vi "ImportCSV.vi"(11 "Settings in":T1={"Name of test"="", "Date"=timestamp(0 s since 1904-01-01), "Location"="", "Template"="", "Soundcard"="", "resolution"=32, "Sampling rate"=48000, "Ch1 Gain "=25.0, "Ch2 Gain"=10.0, "Sample time (s)"=0.3, "Pre-trigger (s)"=0.01, "Hammer Threshold"=10.0, "Positions"=12, "Taps/Position"=5, "Set Names"="", "Freq resolution"=10.0, "Hammer cutoff"=0.0, "Mic cutoff"=0.0, "Double bounce "=0.0, "Hammer Cal"=10.0, "dB Offset"=0.0, "Accel Cal"=10.0, "Vibrometer Cal"=0.0, "Mic Cal"=0.0, "Output"=2, "Voltage Cal"=1.0, "Vibrometer Port"="ASRL27::INSTR", "Range"=4, "High Pass"=2, "Bandwidth"=4, "X Range"=[], "Y Range"=[], "dB Spread"=0.0, "Trigger"=0, "Ch_1"=25, "Ch_2"=25, "flip?"=FALSE, "60Hz"=FALSE, "Time offset"=0.0, "Piezo Cal"=1.0, "Default Notes"=""} {"Ch_2" min=1 step=1; "Ch_1" min=1 max=100 step=1; "Trigger" items=["Hammer (force)", "Self-tap", "Spacebar"]; "Bandwidth" items=["1 kHz"=1, "5 kHz"=5, "10 kHz"=10, "25 kHz"=25, "50 kHz"=50, "100 kHz"=100]; "High Pass" items=["Off", "13 Hz", "104 Hz"]; "Range" items=["10 mm/s"=1, "20 mm/s"=2, "50 mm/s"=5, "100 mm/s"=10, "200 mm/s"=20, "500 mm/s"=50, "1 m/s"=100, "2 m/s"=200]; "Output" items=["Accelerometer", "Speed (from acceleration)", "Microphone", "Vibrometer", "Piezo"]; "Voltage Cal" format="%#_13g"; "Ch2 Gain" format="%#_13g"; "Ch1 Gain" format="%#_13g"; "Double bounce" min=0.0; "Mic cutoff" min=0.0 format="%#_4g"; "Hammer cutoff" min=0.0 format="%#_4g"; "Freq resolution" min=0.0; "Pre-trigger (s)" format="%#_13g"; "Date" format="%<%H:%M\n%d/%m/%y>T"; "resolution" items=["16 bit"=16, "24 bit"=24, "32 bit"=32]; "Sampling rate" items=["22050 samp/s"=22050, "44100 samp/s"=44100, "48000 samp/s"=48000]}) -> ()   [LabVIEW 2022 SP3]
uses:
  PreferencesControl.ctl
  <vilib>/Utility/error.llb/Trim Whitespace One-Sided.vi
panel:
  out "trf":cluster{dbl, dbl, cdb[]}[](array[cluster])
  in  "Tab Control":enum32{"Intro", "Params", "Settings", "Saving"}(tab)
  in  "delimiter":u16(ring) items=["tab", "comma"]
  in  "Save Button":bool
  in  "Instrument Name":string(combo)
  in  "CSV Path":path
  out "FRF":cluster{"x0":dbl, "df":dbl, dbl[]}[](graph)
  out "text":string
  in  "skip first N lines":i32=1
  in  "Back":bool
  out "Slide":u8(slide) scale=0.0..100.0
  out "Info":string
  # "Welcome To The CSV Translator"
  # "This will translate a csv file into the Obie format"
  # "1. Select a file\nHit the folder button or drag a file on"
  # "2. Translate the data\nMake sure the data looks good\n(I assume that the data is evenly sampled\nand that column 1 is time, 2 is real component of pressure\n3 is the complex component, 4 is time, 5 is real,...)"
  # "3. Save as an instrument\nAdd to an existing or create a new instrument"
  # "4. Repeat or Close\nOpen a new file or close the window"
  # "Hz"
  # "dB"
  # "dB"
  # "sec"
  # "sec"
  # "mV/Pa"
  # "mV/m/s2"
  # "mV/mm/s"
  # "V/N"
  # "sec"
  # "sec"
  # "mV/N"
  # "a.u."
  # "a.u."
  # "sec"
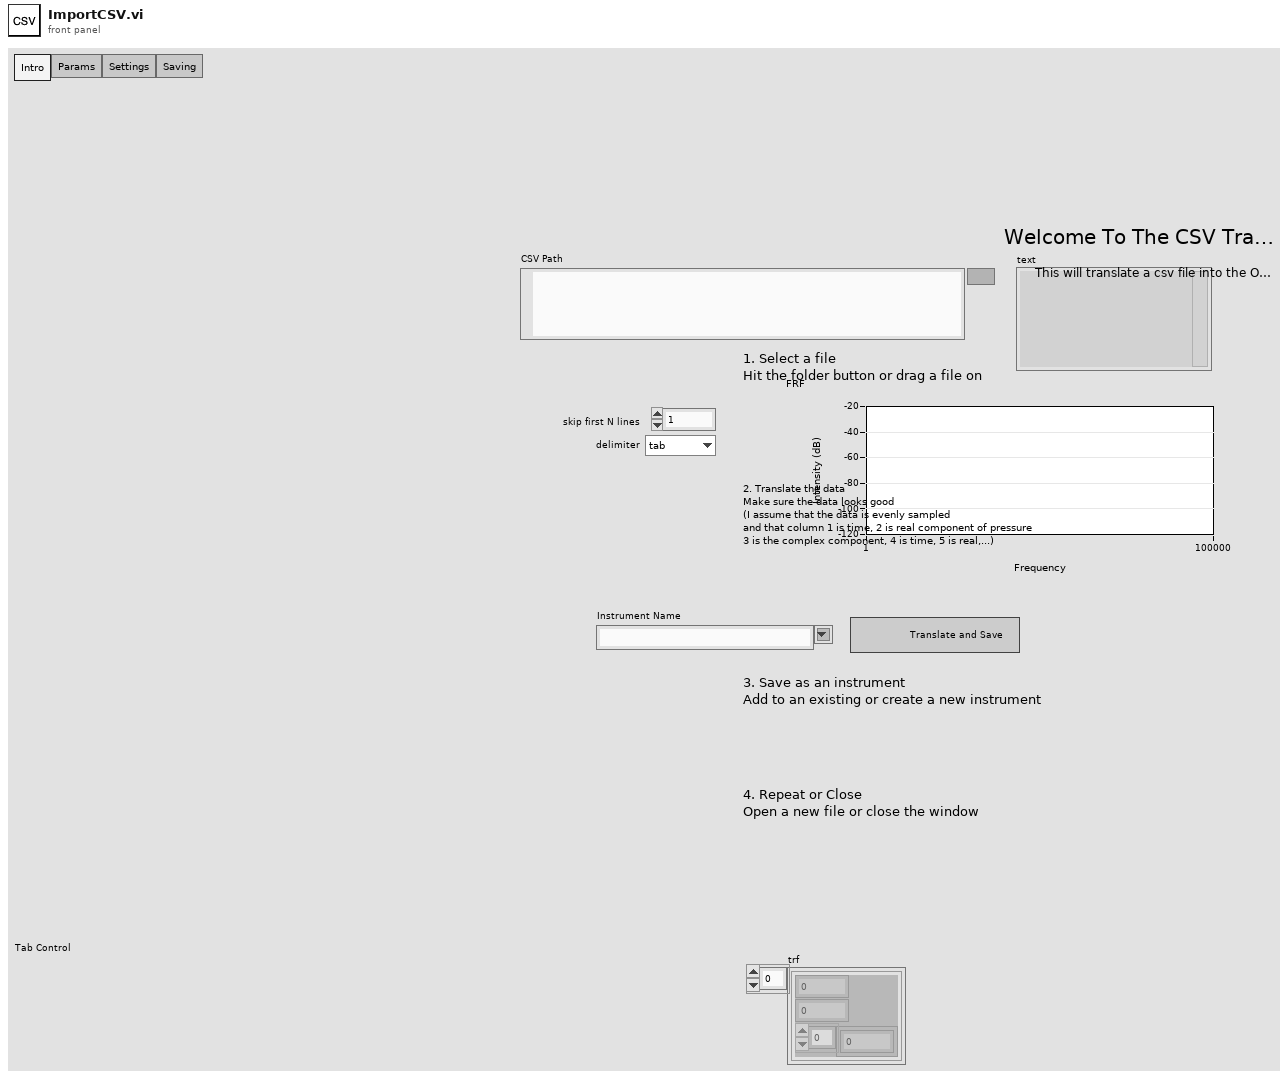
[diagram p1: front panel]
types:
  T1 = typedef "PreferencesControl.ctl" = cluster{"Name of test":string, "Date":timestamp, "Location":string, "Template":string, "Soundcard":string, "resolution":u16, "Sampling rate":u16, "Ch1 Gain ":dbl, "Ch2 Gain":dbl, "Sample time (s)":dbl, "Pre-trigger (s)":dbl, "Hammer Threshold":dbl, "Positions":i16, "Taps/Position":i16, "Set Names":string, "Freq resolution":dbl, "Hammer cutoff":dbl, "Mic cutoff":dbl, "Double bounce ":dbl, "Hammer Cal":dbl, "dB Offset":dbl, "Accel Cal":dbl, "Vibrometer Cal":dbl, "Mic Cal":dbl, "Output":u16, "Voltage Cal":dbl, "Vibrometer Port":refnum<visa-resource-name>, "Range":u16, "High Pass":u16, "Bandwidth":u16, "X Range":cluster{"Minimum":dbl, "Maximum":dbl, "Increment":dbl, "Minor Increment":dbl, "Start":dbl}[], "Y Range":cluster{"Minimum":dbl, "Maximum":dbl, "Increment":dbl, "Minor Increment":dbl, "Start":dbl}[], "dB Spread":dbl, "Trigger":u16, "Ch_1":u8, "Ch_2":u8, "flip?":bool, "60Hz":bool, "Time offset":dbl, "Piezo Cal":dbl, "Default Notes":string}
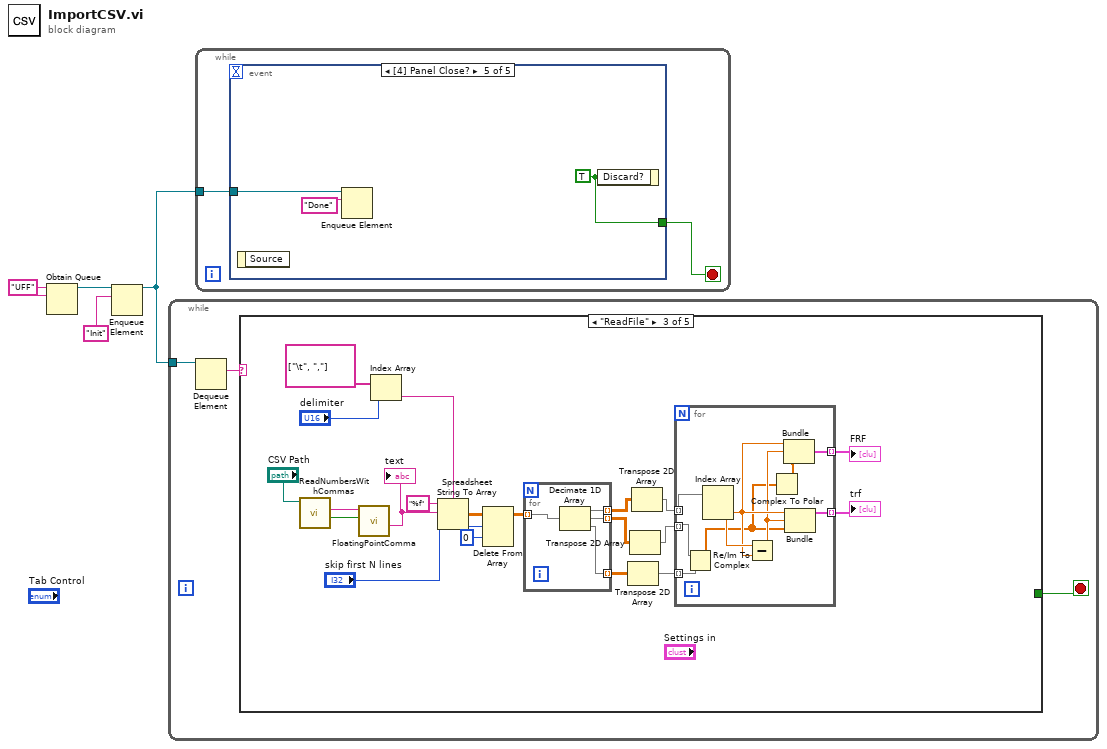
[diagram p0: block diagram]
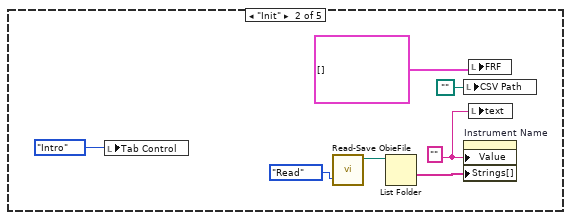
[diagram p3: hidden frame]
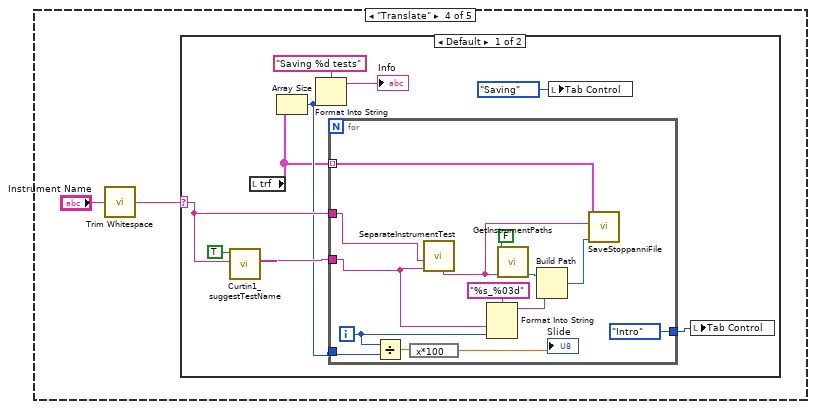
[diagram p4: hidden frame]
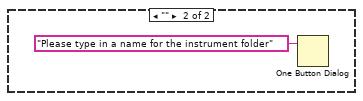
[diagram p5: hidden frame]
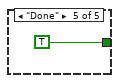
[diagram p6: hidden frame]
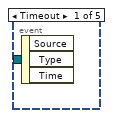
[diagram p7: hidden frame]
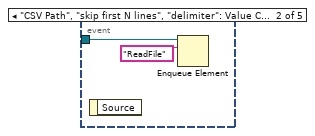
[diagram p8: hidden frame]
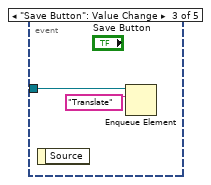
[diagram p9: hidden frame]
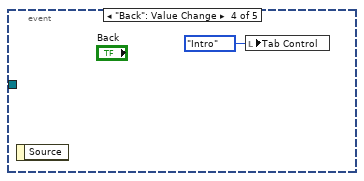
[diagram p10: hidden frame]
diagram:
  w4 = "UFF" ("name (unnamed)")
  n1 = Obtain Queue(name (unnamed)=w4, element data type=w4) -> (queue out=w1:refnum<queue>)  [unwired: 3 in, 2 out]
  n2 = Enqueue Element(queue=w1, element="Init") -> (queue out=w2:refnum<queue>)  [unwired: 2 in, 2 out]
  n3 = while {
    tunnel: w2 -> [w7]
    stop <- w5 stop-if-true
    n4 = Dequeue Element(queue=w7) -> (element=w6:string)  [unwired: 2 in, 3 out]
    n5 = case shown="\"ReadFile\"" w6 {
      tunnel: [_ _ _ _ TRUE ("Discard?")] -> w5
      frame Default {
      }
      frame "Init" {
        w10 = "" ("Value (Signaling)")
        n6 = local write "Tab Control"(enum32{"Intro", "Params", "Settings"}."Intro" ("Tab Control")) -> ()
        n7 = call "Read-Save ObieFile.vi"("Task"=enum16{"Save", "Read"}."Read") -> ("DataPath Out"=w12:path)  [unwired: 8 in, 2 out]
        n8 = List Folder(path=w12) -> (folder names=w11:string[])  [unwired: 3 in, 3 out]
        n9 = local write "CSV Path"(path "" ("CSV Path")) -> ()
        n10 = property on="Instrument Name" class="CmbBox"("Value"=w10, "Strings[]"=w11) -> ()  [unwired: 2 in, 2 out]
        n11 = local write "FRF"(cluster{"x0":dbl, "df":dbl, dbl[]}[] [] ("FRF")) -> ()
        n12 = local write "text"(w10) -> ()
      }
      frame "ReadFile" {
        n13 = call "ReadNumbersWithCommas.vi"("file (use dialog)"="CSV Path") -> ("comma?"=w15:bool, "text"=w17:string)  [unwired: 7 in, 2 out]
        n14 = call "FloatingPointComma.vi"("Comma?"=w15, "String In"=w17) -> ("fixed"=w16:string)  [unwired: 8 in, 1 out]
        "text" <- w16
        n15 = Index Array(array=string[] ["\t", ","], index="delimiter") -> (element=w22:string)
        n16 = Spreadsheet String To Array(delimiter (Tab)=w22, format string="%f", spreadsheet string=w16) -> (array=w33:dbl[][])  [unwired: 1 in]
        n17 = Delete From Array(array=w33, length="skip first N lines", index (row)=0) -> (array with subset deleted=w27:dbl[][])  [unwired: 1 in, 1 out]
        n18 = for {
          tunnel: w27 -> [w48] mode=indexing
          tunnel: [w47] -> w32 mode=indexing
          tunnel: [w46] -> w31 mode=indexing
          tunnel: [w45] -> w21 mode=indexing
          n19 = Decimate 1D Array(w48) -> (w47:dbl[], w46:dbl[], w45:dbl[])
        }
        n20 = Transpose 2D Array(2D array=w21) -> (transposed array=w20:dbl[][])
        n21 = Transpose 2D Array(2D array=w31) -> (transposed array=w29:dbl[][])
        n22 = Transpose 2D Array(2D array=w32) -> (transposed array=w30:dbl[][])
        n23 = for {
          tunnel: w30 -> [w43] mode=indexing
          tunnel: w29 -> [w40] mode=indexing
          tunnel: [w44] -> w28 mode=indexing
          tunnel: w20 -> [w41] mode=indexing
          tunnel: [w37] -> w19 mode=indexing
          n24 = Re/Im To Complex(1:w41, 2:w40) -> (0:w36:cdb[])
          n25 = Index Array(array=w43) -> (element #1=w39:dbl, element #2=w42:dbl)  [unwired: 2 in]
          n26 = Subtract(x=w42, y=w39) -> (x-y=w38:dbl)
          n27 = Complex To Polar(r * e^(i*theta)=w36) -> (r=w35:dbl[])  [unwired: 1 out]
          n28 = Bundle(w39, w38, w35) -> (w37:cluster{dbl, dbl, dbl[]})  [unwired: 1 in]
          n29 = Bundle(w39, w38, w36) -> (w44:cluster{dbl, dbl, cdb[]})  [unwired: 1 in]
        }
        "FRF" <- w19
        "trf" <- w28
      }
      frame "Translate" {
        n30 = call <vilib>:"Trim Whitespace.vi"("string"="Instrument Name") -> ("trimmed string"=w49:string)  [unwired: 1 in]
        n31 = case shown="Default" w49 {
          selector: w49 -> [w58 _]
          frame Default {
            n32 = call "Curtin1_suggestTestName.vi"("instrument"=w58, "Build?"=TRUE) -> ("Suggested Test"=w56:string)  [unwired: 9 in]
            n33 = local read "trf"() -> (w51:cluster{dbl, dbl, cdb[]}[])
            n34 = Array Size(array=w51) -> (size(s)=w54:i32)
            n35 = Format Into String(format string="Saving %d tests", w54) -> (resulting string=→"Info":string)  [unwired: 2 in, 1 out]
            n36 = for {
              tunnel: w58 -> [w69]
              tunnel: w56 -> [w66]
              tunnel: w54 -> [w64]
              tunnel: [enum32{"Intro", "Params", "Settings", "Saving"}."Intro" ("Tab Control")] -> w52
              tunnel: w51 -> [w60] mode=indexing
              i -> [w65]
              n37 = Divide(x=w65, y=w64) -> (x/y=w63:dbl)
              n38 = expression code="x*100"(w63) -> (→"Slide":dbl)
              n39 = call "SeparateInstrumentTest.vi"("test in"=w66, "Instrument in"=w69) -> ("Instrument -- test out"=w72:string)  [unwired: 5 in, 4 out]
              n40 = Format Into String(format string="%s_%03d", w66, w65) -> (resulting string=w67:string)  [unwired: 2 in, 1 out]
              n41 = call "GetInstrumentPaths.vi"("Instrument"=w72, "Build?"=FALSE) -> ("Path To Raw Folder"=w71:path)  [unwired: 5 in, 4 out]
              n42 = Build Path(base path=w71, name or relative path=w67) -> (appended path=w70:path)
              n43 = call "SaveStoppanniFile.vi"("Last Path"=w70, "Inst:Test Name"=w72, "Complex FRF"=w60) -> ()  [unwired: 8 in, 1 out]
            }
            n44 = local write "Tab Control"(enum32{"Intro", "Params", "Settings", "Saving"}."Saving" ("Tab Control")) -> ()
            n45 = local write "Tab Control"(w52) -> ()
          }
          frame "" {
            n46 = One Button Dialog(message="Please type in a name for the instrument folder") -> ()  [unwired: 1 in, 1 out]
          }
        }
      }
      frame "Done" {
      }
    }
  }
  n47 = while {
    tunnel: w2 -> [w77]
    stop <- w76 stop-if-true
    n48 = event shown="[4] Panel Close?" {
      selector: _ -> [_ _ _ _ _]
      dyn-events: _ -> [_ _ _ _ _]
      timeout: _ -> [_ _ _ _ _]
      tunnel: w77 -> [_ w79 w81 _ w83]
      tunnel: [_ _ _ _ w85] -> w76
      event Timeout {
        n49 = event-data() -> ()  [unwired: 1 in, 3 out]
      }
      event "CSV Path", "skip first N lines", "delimiter": Value Change {
        n50 = event-data() -> ()  [unwired: 1 in, 1 out]
        n51 = Enqueue Element(queue=w79, element="ReadFile") -> ()  [unwired: 2 in, 3 out]
      }
      event "Save Button": Value Change {
        n52 = event-data() -> ()  [unwired: 1 in, 1 out]
        n53 = Enqueue Element(queue=w81, element="Translate") -> ()  [unwired: 2 in, 3 out]
      }
      event "Back": Value Change {
        n54 = event-data() -> ()  [unwired: 1 in, 1 out]
        n55 = local write "Tab Control"(enum32{"Intro", "Params", "Settings"}."Intro" ("Tab Control")) -> ()
      }
      event Panel Close? {
        w85 = TRUE ("Discard?")
        n56 = event-data() -> ()  [unwired: 1 in, 1 out]
        n57 = Enqueue Element(queue=w83, element="Done") -> ()  [unwired: 2 in, 3 out]
        n58 = event-data("Discard?"=w85) -> ()  [unwired: 1 in, 1 out]
      }
    }
  }
